vi "GSE 350 Parse Data Stream.vi"(5 "Data Stream":string, 11 "Error In":errorcluster) -> (4 "Data Array":string[][](array[string]), 6 "Tare Weight":dbl, 8 "Net Weight":dbl, 10 "Gross Weight":dbl, 14 "Match Found!":bool, 15 "Error Out":errorcluster)   [LabVIEW 2020]
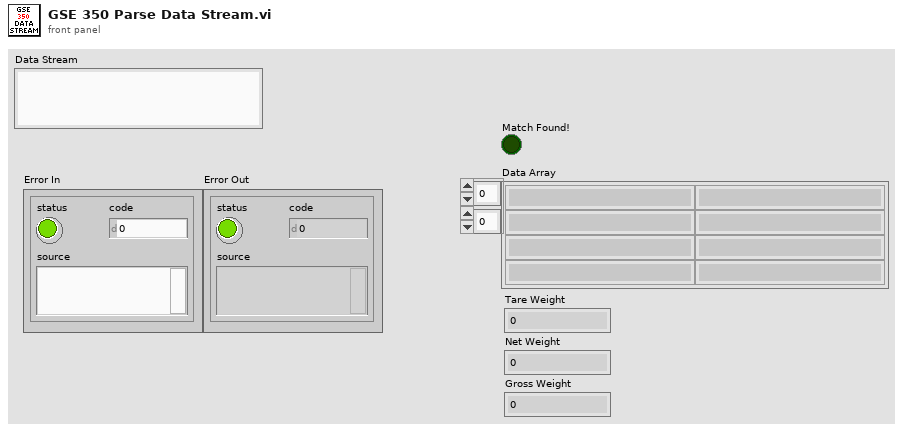
[diagram p1: front panel]
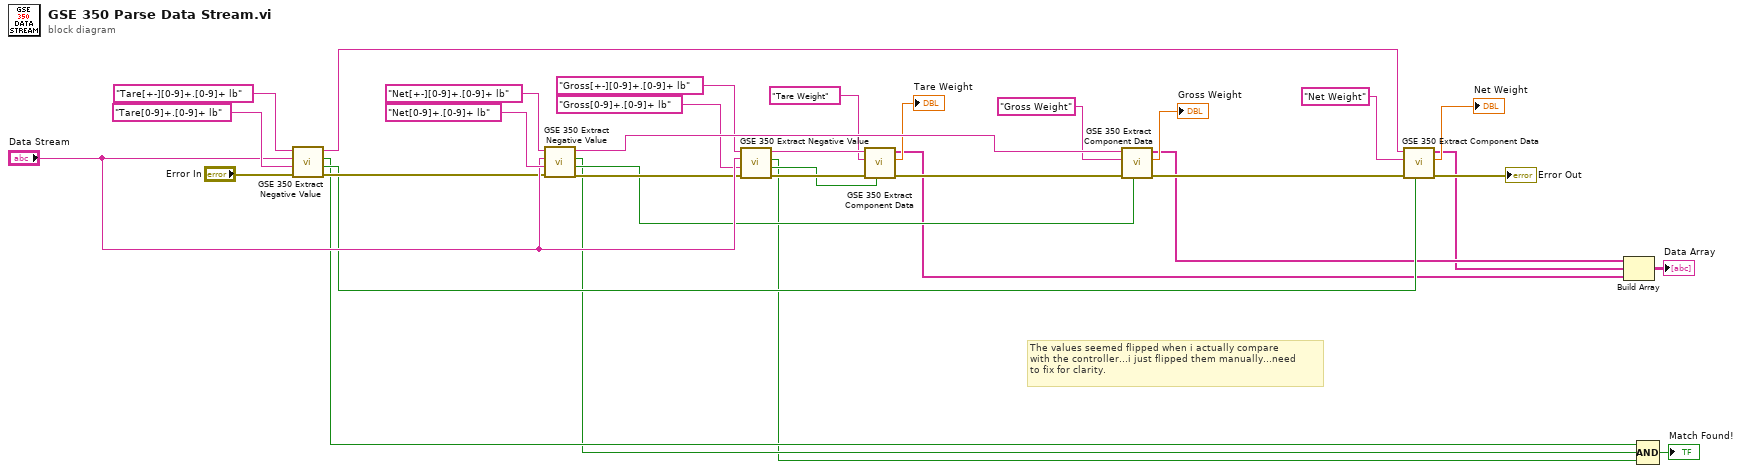
[diagram p0: block diagram]
diagram:
  # "The values seemed flipped when i actually compare\nwith the controller...i just flipped them manually...need \nto fix for clarity."
  n1 = call "GSE 350 Extract Negative Value.vi"("Error In"="Error In", "Regular Expression Search"="Tare[0-9]+.[0-9]+ lb" ("regular expression"), "Full String"="Data Stream", "Expression With Negative Search"="Tare[+-][0-9]+.[0-9]+ lb" ("regular expression")) -> ("Error Out"=w23:errorcluster, "Negative Number?"=w14:bool, "Found Match"=w4:bool, "Output Match"=w31:string)  [unwired: 4 in]
  n2 = call "GSE 350 Extract Negative Value.vi"("Error In"=w23, "Regular Expression Search"="Net[0-9]+.[0-9]+ lb" ("regular expression"), "Full String"="Data Stream", "Expression With Negative Search"="Net[+-][0-9]+.[0-9]+ lb" ("regular expression")) -> ("Error Out"=w22:errorcluster, "Negative Number?"=w15:bool, "Found Match"=w3:bool, "Output Match"=w28:string)  [unwired: 4 in]
  n3 = call "GSE 350 Extract Negative Value.vi"("Error In"=w22, "Regular Expression Search"="Gross[0-9]+.[0-9]+ lb" ("regular expression"), "Full String"="Data Stream", "Expression With Negative Search"="Gross[+-][0-9]+.[0-9]+ lb" ("regular expression")) -> ("Error Out"=w21:errorcluster, "Negative Number?"=w16:bool, "Found Match"=w2:bool, "Output Match"=w24:string)  [unwired: 4 in]
  n4 = call "GSE 350 Extract Component Data.vi"("Negative Number"=w16, "Error In"=w21, "Title"="Tare Weight", "Data Stream"=w24) -> ("Error Out"=w20:errorcluster, "Weight"=→"Tare Weight":dbl, "Array"=w5:string[])  [unwired: 5 in]
  n5 = call "GSE 350 Extract Component Data.vi"("Negative Number"=w15, "Error In"=w20, "Title"="Gross Weight", "Data Stream"=w28) -> ("Error Out"=w19:errorcluster, "Weight"=→"Gross Weight":dbl, "Array"=w7:string[])  [unwired: 5 in]
  n6 = call "GSE 350 Extract Component Data.vi"("Negative Number"=w14, "Error In"=w19, "Title"="Net Weight", "Data Stream"=w31) -> ("Error Out"=→"Error Out":errorcluster, "Weight"=→"Net Weight":dbl, "Array"=w6:string[])  [unwired: 5 in]
  n7 = Build Array(w7, w6, w5) -> (→"Data Array":string[][])
  n8 = Compound Arithmetic op=AND(w4, w3, w2) -> (→"Match Found!":bool)
